vi "Klinger Control.vi"(8 "error in":errorcluster, 9 "PosDem":dbl caption="Allez à" min=-7999999.9 max=7999999.9 step=0.1 format="%.1f", 10 "Relatif":bool caption="Relatif/Absolu\n(Absolu)", 11 "Axe":u8(ring)=3 items=["W", "X", "Y", "Z"]) -> (0 "error out":errorcluster, 1 "Position":dbl min=-7999999.9 max=7999999.9 step=0.1 format="%.1f", 2 "NLimit":bool caption="Limite -", 3 "PLimit":bool caption="Limite +", 5 "Axe out":u8(ring)=3 caption="Axe" items=["W", "X", "Y", "Z"])   [LabVIEW 2010]
doc: "Ce Vi est une interface de contrôle complète d'où on peut effectué les diverse fonction du contrôlleur Klinger"
uses:
  <vilib>/Utility/error.llb/DialogType.ctl
  <userlib>/Klinger/Klinger Lib.llb/Klinger ConvUnitSgl.vi
  <userlib>/Klinger/Klinger Lib.llb/Klinger ConvUnitArr.vi
panel:
  in  "ReadPos":bool
  in  "ModParam":bool
  out "Nom de l'axe":string
  out "CorrParams":T1={"CorrActive"=FALSE, "ErreurLim"=0.1, "NbrEssais"=3} caption="Paramètres de \ncorrection de position" {"NbrEssais" min=1 max=5 step=1; "ErreurLim" min=0.0 max=10.0 step=0.1 format="%#.1f"}
  out "Adresse":string
  in  "Unit":u8(ring) caption="Unité:" items=["Pas", "mm", "ps", "Degré (°)"]
  in  "Default":bool
  in  "Zero":bool
  in  "Accel":sgl=0.4 caption="Accélération" min=0.1 max=2 step=0.1 format="%#.1f"
  in  "Speed Type":enum32{"Pas/Seconde", "ms/Pas"}(radio)
  in  "Vitesse":i32=800 min=32 max=4000 step=1 format="%#.0f"
  in  "stop":bool
  in  "RAZ":bool
  in  "Origine":bool
  out "PosErreur":dbl caption="Erreur de\nPositionnement" min=-7999999.9 max=7999999.9 step=0.1 format="%.1f"
  out "Indcomm":string caption="Terminal Indicateur"
  out "Pos Init":dbl caption="Position Initiale" min=-7999999.9 max=7999999.9 step=0.1 format="%.1f"
  out "Moving":bool caption="Déplacement\nen cours"
  out "Erreur":bool
  # "Commandes"
  # "Paramètres"
  # "Sec"
  # "Relatif"
  # "Absolu"
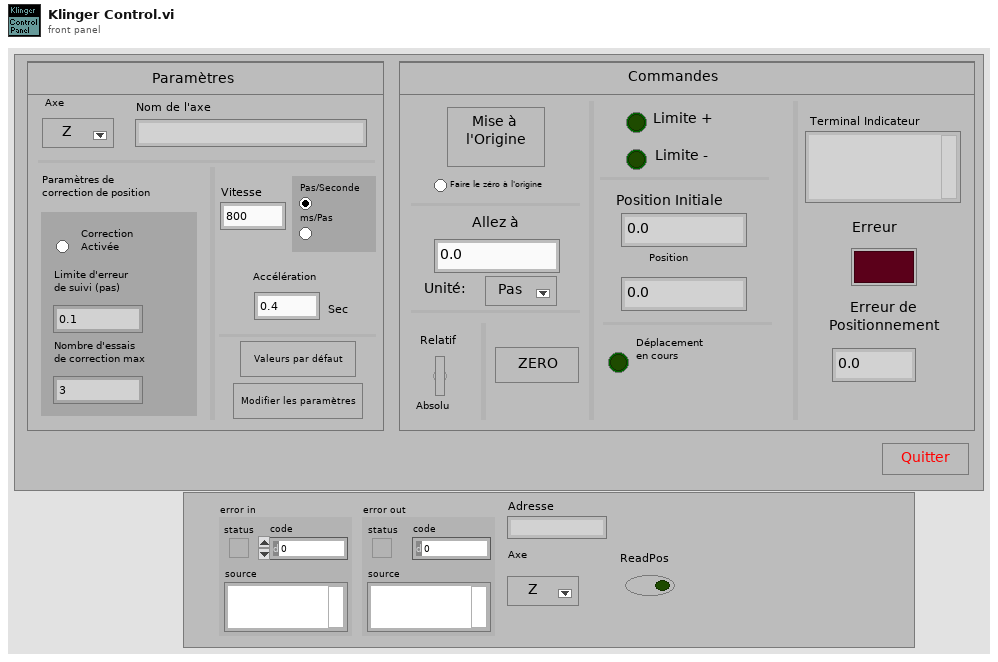
[diagram p1: front panel]
types:
  T1 = cluster{"CorrActive":bool, "ErreurLim":dbl, "NbrEssais":i32}
  T2 = cluster{"Minimum":dbl, "Maximum":dbl, "Increment":dbl}
  T3 = typedef "DialogType.ctl" = u16
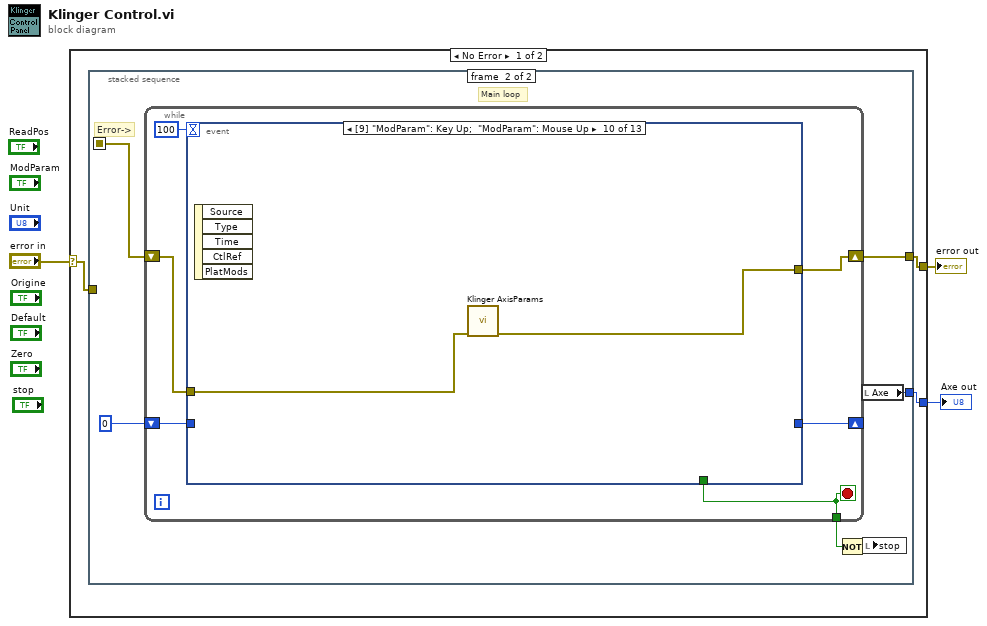
[diagram p0: block diagram]
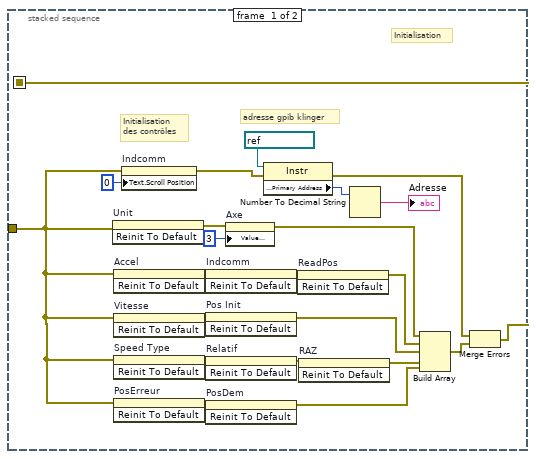
[diagram p2: hidden frame]
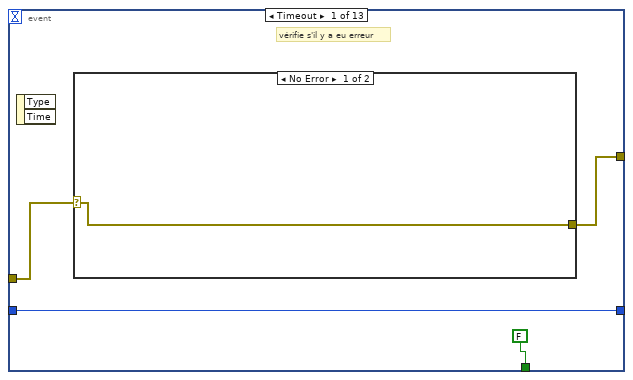
[diagram p3: hidden frame]
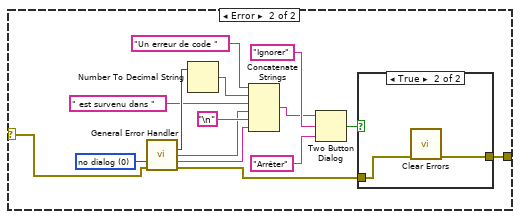
[diagram p4: hidden frame]
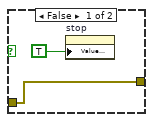
[diagram p5: hidden frame]
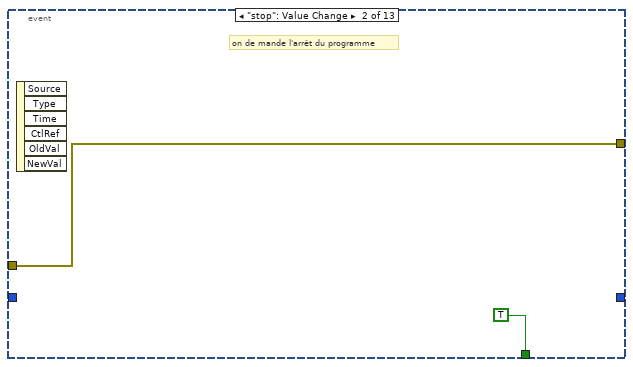
[diagram p6: hidden frame]
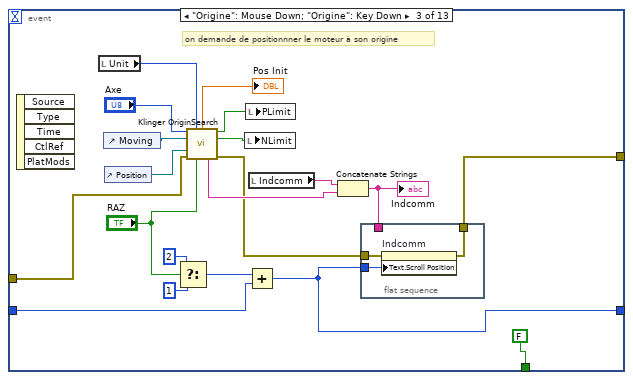
[diagram p7: hidden frame]
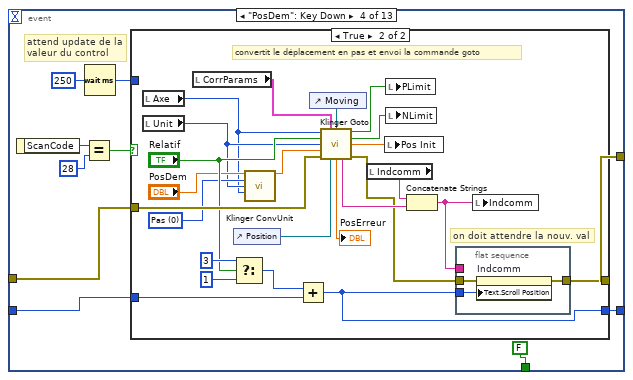
[diagram p8: hidden frame]
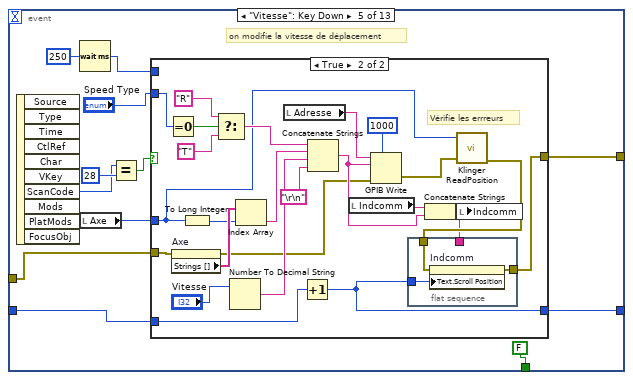
[diagram p10: hidden frame]
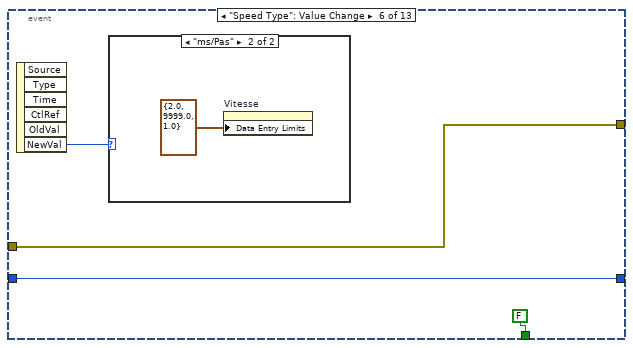
[diagram p12: hidden frame]
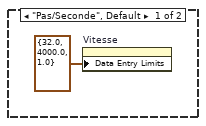
[diagram p13: hidden frame]
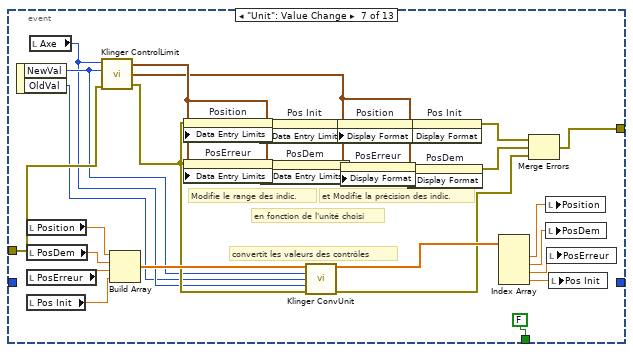
[diagram p14: hidden frame]
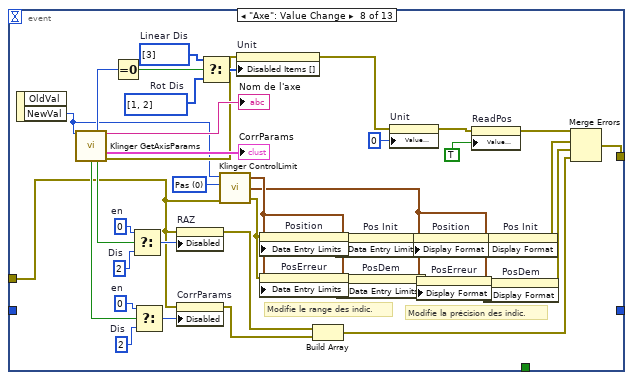
[diagram p15: hidden frame]
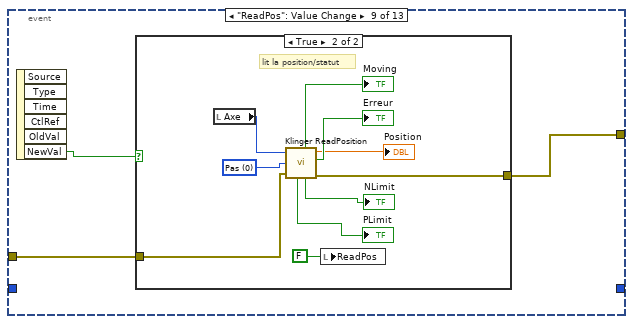
[diagram p16: hidden frame]
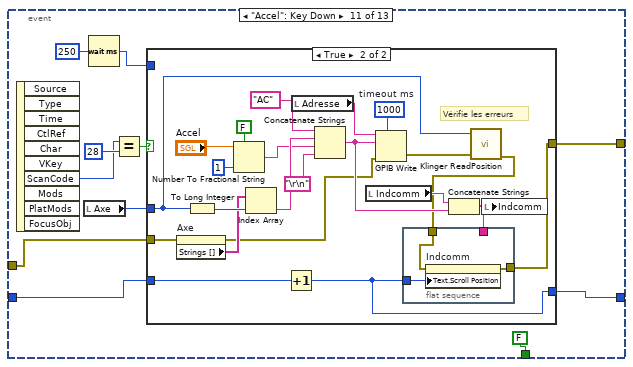
[diagram p18: hidden frame]
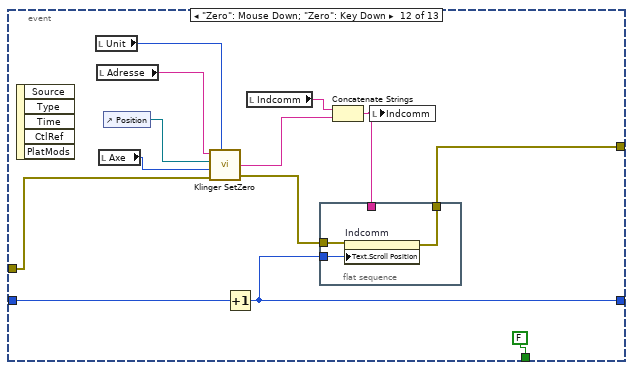
[diagram p20: hidden frame]
diagram:
  n1 = case shown="No Error" "error in" {
    selector: "error in" -> [w5 w345]
    tunnel: [w6 w345] -> w3
    tunnel: [w4 u8 0 ("Axe")] -> w1
    frame No Error {
      n2 = stacked-sequence {
        seq-local: [w7 _] -> [_ w33]
        tunnel: [_ w34] -> w6
        tunnel: w5 -> [w15 _]
        tunnel: [_ w29] -> w4
        frame #0 {
          # "adresse gpib klinger"
          # "Initialisation\ndes contrôles"
          # "Initialisation"
          n3 = invoke on="Unit" class="Ring (strict)" method="Reinit To Default"(error in=w15) -> (error out=w8:errorcluster)  [unwired: 2 in, 2 out]
          n4 = invoke on="Accel" class="DigNum (strict)" method="Reinit To Default"(error in=w15) -> (error out=w24:errorcluster)  [unwired: 2 in, 2 out]
          n5 = invoke on="Vitesse" class="DigNum (strict)" method="Reinit To Default"(error in=w15) -> (error out=w23:errorcluster)  [unwired: 2 in, 2 out]
          n6 = invoke on="Speed Type" class="RadioBtnsControl (strict)" method="Reinit To Default"(error in=w15) -> (error out=w22:errorcluster)  [unwired: 2 in, 2 out]
          n7 = invoke on="PosErreur" class="DigNum (strict)" method="Reinit To Default"(error in=w15) -> (error out=w17:errorcluster)  [unwired: 2 in, 2 out]
          n8 = property on="Indcomm" class="Str"(error in=w15, "Text.Scroll Position"=u32 0) -> (error out=w25:errorcluster)  [unwired: 1 in, 1 out]
          n9 = invoke on="Indcomm" class="Str" method="Reinit To Default"(error in=w24) -> (error out=w10:errorcluster)  [unwired: 2 in, 2 out]
          n10 = invoke on="Pos Init" class="DigNum (strict)" method="Reinit To Default"(error in=w23) -> (error out=w11:errorcluster)  [unwired: 2 in, 2 out]
          n11 = invoke on="Relatif" class="Bool (strict)" method="Reinit To Default"(error in=w22) -> (error out=w16:errorcluster)  [unwired: 2 in, 2 out]
          n12 = invoke on="PosDem" class="DigNum (strict)" method="Reinit To Default"(error in=w17) -> (error out=w21:errorcluster)  [unwired: 2 in, 2 out]
          n13 = property on="Axe" class="Ring (strict)"(error in=w8, "Value (Signaling)"=u8 3) -> (error out=w12:errorcluster)  [unwired: 1 in, 1 out]
          n14 = property class="Instr"(reference=refnum<visa-resource-name> "KLINGER", error in=w25) -> (error out=w19:errorcluster, "GPIB Settings:Primary Address"=w28:u16)  [unwired: 1 out]
          n15 = invoke on="ReadPos" class="Boolean (strict)" method="Reinit To Default"(error in=w10) -> (error out=w9:errorcluster)  [unwired: 2 in, 2 out]
          n16 = invoke on="RAZ" class="Bool (strict)" method="Reinit To Default"(error in=w16) -> (error out=w18:errorcluster)  [unwired: 2 in, 2 out]
          n17 = Number To Decimal String(number=w28) -> (decimal integer string=→"Adresse":string)  [unwired: 1 in]
          n18 = Build Array(w12, w9, w11, w18, w21) -> (w20:errorcluster[])
          n19 = Merge Errors(w19, w20) -> (w7:errorcluster)
        }
        frame #1 {
          # "Main loop"
          # "Error->"
          n20 = while {
            shift-right: [w36] -> w34
            shift-left: w33 -> [w39]
            shift-right: [w37] -> _
            shift-left: u32 0 ("Text.Scroll Position") -> [w38]
            tunnel: [w35] -> w31
            stop <- w35 stop-if-true
            n21 = event shown="[9] \"ModParam\": Key Up;  \"ModParam\": Mouse Up" {
              selector: _ -> [_ _ _ _ _ _ _ _ _ _ _ _ _]
              dyn-events: _ -> [_ _ _ _ _ _ _ _ _ _ _ _ _]
              timeout: 100 -> [_ _ _ _ _ _ _ _ _ _ _ _ _]
              tunnel: w39 -> [w41 w65 w77 w97 w136 w172 w188 w211 w244 w258 w266 w307 w334]
              tunnel: [w43 w65 w73 w93 w132 w172 w197 w217 w243 w257 w263 w300 w315] -> w36
              tunnel: w38 -> [w44 _ w82 w96 w135 w171 _ _ _ _ w262 w306 w331]
              tunnel: [w44 _ w81 w95 w134 w171 _ _ _ _ w265 w305 w317] -> w37
              tunnel: [FALSE TRUE FALSE FALSE FALSE FALSE FALSE _ _ _ FALSE FALSE FALSE] -> w35
              event Timeout {
                # "vérifie s'il y a eu erreur"
                n22 = event-data() -> ()  [unwired: 1 in, 2 out]
                n23 = case shown="No Error" w41 {
                  selector: w41 -> [w45 w46]
                  tunnel: [w45 w47] -> w43
                  frame No Error {
                  }
                  frame Error {
                    w57 = T3 0 items=["no dialog", "OK message", "continue or stop message", "OK message + warnings", "continue/stop + warnings"] ("type of dialog (OK msg:1)")
                    n24 = call <vilib>:"General Error Handler.vi"("type of dialog (OK msg:1)"=w57, "error in (no error)"=w46) -> ("code out"=w53:i32, "source out"=w52:string, "message"=w50:string, "error out"=w48:errorcluster)  [unwired: 9 in, 1 out]
                    n25 = Number To Decimal String(number=w53) -> (decimal integer string=w54:string)  [unwired: 1 in]
                    n26 = Concatenate Strings("Un erreur de code " ("string"), w54, " est survenu dans " ("string"), w52, "\n", w50) -> (w49:string)
                    n27 = Two Button Dialog(message=w49, 1:"Arrêter" ("F button name (\"Cancel\")"), 2:"Ignorer" ("T button name (\"OK\")")) -> (T button?=w60:bool)
                    n28 = case shown="True" w60 {
                      tunnel: w48 -> [w62 w64]
                      tunnel: [w62 w63] -> w47
                      frame False {
                        n29 = property on="stop" class="Bool (strict)"("Value (Signaling)"=TRUE) -> ()  [unwired: 2 in, 2 out]
                      }
                      frame True {
                        n30 = call <vilib>:"Clear Errors.vi"("error in (no error)"=w64) -> ("error out"=w63:errorcluster)  [unwired: 6 in]
                      }
                    }
                  }
                }
              }
              event "stop": Value Change {
                # "on de mande l'arrêt du programme"
                n31 = event-data() -> ()  [unwired: 1 in, 6 out]
              }
              event "Origine": Mouse Down; "Origine": Key Down {
                # "on demande de positionnner le moteur à son origine"
                n32 = event-data() -> ()  [unwired: 1 in, 5 out]
                n33 = local read "Unit"() -> (w67:u8)
                n34 = control-ref of="Moving"() -> (w83:refnum<vi>)
                n35 = control-ref of="Position"() -> (w84:refnum<vi>)
                n36 = Select(t=u32 2 ("x+y"), s="RAZ", f=u32 1 ("x+y")) -> (s? t:f=w80:u32)
                n37 = call <userlib>:"Klinger OriginSearch.vi"("Axe"="Axe", "UnitDem"=w67, "Moving Ref"=w83, "Position Ref"=w84, "error in"=w77, "Set as Zero"="RAZ") -> ("Pos Init"=→"Pos Init":dbl, "PLimit"=w85:bool, "NLimit"=w86:bool, "Indcomm"=w75:string, "error out"=w74:errorcluster)  [unwired: 3 in, 2 out]
                n38 = local write "NLimit"(w86) -> ()
                n39 = local write "PLimit"(w85) -> ()
                n40 = Add(x=w80, y=w82) -> (x+y=w81:u32)
                n41 = local read "Indcomm"() -> (w76:string)
                n42 = Concatenate Strings(w76, w75) -> (w69:string)
                "Indcomm" <- w69
                n43 = flat-sequence {
                  tunnel: w81 -> [w89]
                  tunnel: w69 -> [_]
                  tunnel: w74 -> [w88]
                  tunnel: [w87] -> w73
                  frame #0 {
                    n44 = property on="Indcomm" class="Str"(error in=w88, "Text.Scroll Position"=w89) -> (error out=w87:errorcluster)  [unwired: 1 in, 1 out]
                  }
                }
              }
              event "PosDem": Key Down {
                # "attend update de la \nvaleur du control"
                n45 = event-data() -> ("ScanCode"=w94:i16)  [unwired: 1 in]
                n46 = Equal?(x=w94, y=i16 28) -> (x = y?=w98:bool)
                n47 = Wait (ms)(milliseconds to wait=u32 250) -> (millisecond timer value=w91:u32)
                n48 = case shown="True" w98 {
                  tunnel: w97 -> [w100 w123]
                  tunnel: w96 -> [w101 w122]
                  tunnel: [w101 w113] -> w95
                  tunnel: [w100 w114] -> w93
                  tunnel: w91 -> [_ _]
                  frame False {
                  }
                  frame True {
                    w106 = u8 0 items=["Pas", "mm", "ps"] ("UnitDem")
                    # "convertit le déplacement en pas et envoi la commande goto"
                    # "on doit attendre la nouv. val"
                    n49 = local read "Axe"() -> (w103:u8)
                    n50 = local read "Unit"() -> (w104:u8)
                    n51 = local read "CorrParams"() -> (w102:T1)
                    n52 = control-ref of="Position"() -> (w115:refnum<vi>)
                    n53 = Select(t=u32 3 ("Text.Scroll Position"), s="Relatif", f=u32 1 ("Text.Scroll Position")) -> (s? t:f=w119:u32)
                    n54 = call-poly <userlib>:"Klinger ConvUnit.vi"("ParamAct"="PosDem", "UnitDem"=w106, "UnitAct"=w104, "Axe"=w103) -> ("ParamDem"=w105:dbl)  [unwired: 10 in, 1 out]
                    n55 = Add(x=w119, y=w122) -> (x+y=w113:u32)
                    n56 = control-ref of="Moving"() -> (w118:refnum<vi>)
                    n57 = call <userlib>:"Klinger Goto.vi"("Axe"=w103, "Suivi"=w102, "Moving Ref"=w118, "Relatif"="Relatif", "UnitDem"=w104, "PosDem"=w105, "error in"=w123, "Position Ref"=w115) -> ("PLimit"=w125:bool, "NLimit"=w124:bool, "Pos Init"=w109:dbl, "PosErreur"=→"PosErreur":dbl, "Indcomm"=w116:string, "error out"=w108:errorcluster)  [unwired: 2 out]
                    n58 = local read "Indcomm"() -> (w117:string)
                    n59 = local write "Pos Init"(w109) -> ()
                    n60 = local write "PLimit"(w125) -> ()
                    n61 = local write "NLimit"(w124) -> ()
                    n62 = Concatenate Strings(w117, w116) -> (w112:string)
                    n63 = flat-sequence {
                      tunnel: w113 -> [w128]
                      tunnel: w108 -> [w127]
                      tunnel: [w126] -> w114
                      tunnel: w112 -> [_]
                      frame #0 {
                        n64 = property on="Indcomm" class="Str"(error in=w127, "Text.Scroll Position"=w128) -> (error out=w126:errorcluster)  [unwired: 1 in, 1 out]
                      }
                    }
                    n65 = local write "Indcomm"(w112) -> ()
                  }
                }
              }
              event "Vitesse": Key Down {
                # "on modifie la vitesse de déplacement"
                n66 = event-data() -> ("ScanCode"=w133:i16)  [unwired: 1 in, 9 out]
                n67 = Wait (ms)(milliseconds to wait=u32 250) -> (millisecond timer value=w129:u32)
                n68 = local read "Axe"() -> (w137:u8)
                n69 = Equal?(x=w133, y=i16 28) -> (x = y?=w139:bool)
                n70 = case shown="True" w139 {
                  tunnel: "Speed Type" -> [_ w165]
                  tunnel: w137 -> [_ w148]
                  tunnel: [w142 w146] -> w132
                  tunnel: w136 -> [w142 w154]
                  tunnel: w135 -> [w141 w145]
                  tunnel: [w141 w153] -> w134
                  tunnel: w129 -> [_ _]
                  frame False {
                  }
                  frame True {
                    # "Vérifie les errreurs"
                    n71 = Equal To 0?(x=w165) -> (x = 0?=w164:bool)
                    n72 = property on="Axe" class="Ring (strict)"(error in=w154) -> (error out=w151:errorcluster, "Strings []"=w161:string[])  [unwired: 1 in, 1 out]
                    n73 = To Long Integer(number=w148) -> (32bit integer=w160:i32)
                    n74 = Select(t="R", s=w164, f="T") -> (s? t:f=w162:string)
                    n75 = Number To Decimal String(number="Vitesse") -> (decimal integer string=w157:string)  [unwired: 1 in]
                    n76 = Index Array(array=w161, index=w160) -> (element=w159:string)
                    n77 = local read "Adresse"() -> (w149:string)
                    n78 = Increment(x=w145) -> (x+1=w153:u32)
                    n79 = Concatenate Strings(w162, w159, w157, "\r\n") -> (w156:string)
                    n80 = local read "Indcomm"() -> (w155:string)
                    n81 = GPIB Write(0:w149, 1:w156, 3:w151, 4:1000 ("timeout ms (488.2 global)")) -> (6:w152:errorcluster)  [unwired: 1 in, 1 out]
                    n82 = flat-sequence {
                      tunnel: w153 -> [w169]
                      tunnel: w147 -> [w168]
                      tunnel: [w167] -> w146
                      tunnel: w144 -> [_]
                      frame #0 {
                        n83 = property on="Indcomm" class="Str"(error in=w168, "Text.Scroll Position"=w169) -> (error out=w167:errorcluster)  [unwired: 1 in, 1 out]
                      }
                    }
                    n84 = Concatenate Strings(w155, w156) -> (w144:string)
                    n85 = call <userlib>:"Klinger ReadPosition.vi"("Axe"=w148, "error in"=w152) -> ("error out"=w147:errorcluster)  [unwired: 2 in, 6 out]
                    n86 = local write "Indcomm"(w144) -> ()
                  }
                }
              }
              event "Speed Type": Value Change {
                n87 = event-data() -> ("NewVal"=w173:enum32{"Pas/Seconde", "ms/Pas"})  [unwired: 1 in, 5 out]
                n88 = case shown="\"ms/Pas\"" w173 {
                  frame "Pas/Seconde", Default {
                    n89 = property on="Vitesse" class="DigNum (strict)"("Data Entry Limits"=T2 {"Minimum"=32.0, "Maximum"=4000.0, "Increment"=1.0} ("Data Range")) -> ()  [unwired: 2 in, 2 out]
                  }
                  frame "ms/Pas" {
                    n90 = property on="Vitesse" class="DigNum (strict)"("Data Entry Limits"=T2 {"Minimum"=2.0, "Maximum"=9999.0, "Increment"=1.0} ("Data Range")) -> ()  [unwired: 2 in, 2 out]
                  }
                }
              }
              event "Unit": Value Change {
                # "convertit les valeurs des contrôles"
                # "en fonction de l'unité choisi"
                # "et Modifie la précision des indic."
                # "Modifie le range des indic."
                n91 = event-data() -> ("NewVal"=w178:u8, "OldVal"=w176:u8)  [unwired: 1 in]
                n92 = local read "Position"() -> (w201:dbl)
                n93 = local read "PosDem"() -> (w202:dbl)
                n94 = local read "PosErreur"() -> (w203:dbl)
                n95 = local read "Pos Init"() -> (w200:dbl)
                n96 = local read "Axe"() -> (w177:u8)
                n97 = call <userlib>:"Klinger ControlLimit.vi"("Axe"=w177, "UnitDem"=w178, "error in"=w188) -> ("DataRange"=w186:T2, "FormtPrec"=w185:cluster{"Format":u8, "Precision":u8}, "error out"=w187:errorcluster)  [unwired: 2 in]
                n98 = Build Array(w201, w202, w203, w200) -> (w195:dbl[])
                n99 = property on="Position" class="DigNum (strict)"(error in=w187, "Data Entry Limits"=w186) -> (error out=w184:errorcluster)  [unwired: 1 in, 1 out]
                n100 = property on="PosErreur" class="DigNum (strict)"(error in=w187, "Data Entry Limits"=w186) -> (error out=w183:errorcluster)  [unwired: 1 in, 1 out]
                n101 = property on="Pos Init" class="DigNum (strict)"(error in=w184, "Data Entry Limits"=w186) -> (error out=w179:errorcluster)  [unwired: 1 in, 1 out]
                n102 = property on="PosDem" class="DigNum (strict)"(error in=w183, "Data Entry Limits"=w186) -> (error out=w180:errorcluster)  [unwired: 1 in, 1 out]
                n103 = call-poly <userlib>:"Klinger ConvUnit.vi"("ParamAct"=w195, "UnitDem"=w178, "UnitAct"=w176, "Axe"=w177, "error in"=w187) -> ("ParamDem"=w194:dbl[], "error out"=w189:errorcluster)  [unwired: 9 in]
                n104 = property on="Position" class="DigNum (strict)"(error in=w179, "Display Format"=w185) -> (error out=w182:errorcluster)  [unwired: 1 in, 1 out]
                n105 = property on="PosErreur" class="DigNum (strict)"(error in=w180, "Display Format"=w185) -> (error out=w181:errorcluster)  [unwired: 1 in, 1 out]
                n106 = property on="Pos Init" class="DigNum (strict)"(error in=w182, "Display Format"=w185) -> (error out=w199:errorcluster)  [unwired: 1 in, 1 out]
                n107 = property on="PosDem" class="DigNum (strict)"(error in=w181, "Display Format"=w185) -> (error out=w198:errorcluster)  [unwired: 1 in, 1 out]
                n108 = Index Array(array=w194) -> (element #1=w193:dbl, element #2=w192:dbl, element #3=w191:dbl, element #4=w190:dbl)  [unwired: 4 in]
                n109 = Merge Errors(w199, w198, w189) -> (w197:errorcluster)
                n110 = local write "Position"(w193) -> ()
                n111 = local write "PosDem"(w192) -> ()
                n112 = local write "PosErreur"(w191) -> ()
                n113 = local write "Pos Init"(w190) -> ()
              }
              event "Axe": Value Change {
                w218 = u8 0 items=["Pas", "mm", "ps", "Degré (°)"] ("UnitDem")
                w231 = i32[] [1, 2]  # Rot Dis
                w232 = i32[] [3]  # Linear Dis
                w236 = u8 2  # Dis
                w235 = u8 0  # en
                w238 = u8 2  # Dis
                w239 = u8 0  # en
                # "Modifie la précision des indic."
                # "Modifie le range des indic."
                n114 = event-data() -> ("NewVal"=w209:u8)  [unwired: 1 in, 1 out]
                n115 = call <userlib>:"Klinger GetAxisParams.vi"("Axe"=w209) -> ("TypeMouv"=w230:i32, "Nom de l'axe"=→"Nom de l'axe":string, "CorrParams"=→"CorrParams":T1, "Encodeur"=w237:bool, "MiseàZéro"=w234:bool, "error out"=w210:errorcluster)  [unwired: 7 in, 2 out]
                n116 = Equal To 0?(x=w230) -> (x = 0?=w229:bool)
                n117 = Select(t=w235, s=w234, f=w236) -> (s? t:f=w233:u8)
                n118 = Select(t=w239, s=w237, f=w238) -> (s? t:f=w240:u8)
                n119 = property on="RAZ" class="Bool (strict)"(error in=w211, "Disabled"=w233) -> (error out=w216:errorcluster)  [unwired: 1 in, 1 out]
                n120 = property on="CorrParams" class="Clust (strict)"(error in=w211, "Disabled"=w240) -> (error out=w215:errorcluster)  [unwired: 1 in, 1 out]
                n121 = Select(t=w232, s=w229, f=w231) -> (s? t:f=w228:i32[])
                n122 = call <userlib>:"Klinger ControlLimit.vi"("Axe"=w209, "UnitDem"=w218, "error in"=w211) -> ("DataRange"=w227:T2, "FormtPrec"=w226:cluster{"Format":u8, "Precision":u8}, "error out"=w219:errorcluster)  [unwired: 2 in]
                n123 = property on="Unit" class="Ring (strict)"(error in=w210, "Disabled Items []"=w228) -> (error out=w207:errorcluster)  [unwired: 1 in, 1 out]
                n124 = property on="Position" class="DigNum (strict)"(error in=w219, "Data Entry Limits"=w227) -> (error out=w225:errorcluster)  [unwired: 1 in, 1 out]
                n125 = property on="PosErreur" class="DigNum (strict)"(error in=w219, "Data Entry Limits"=w227) -> (error out=w224:errorcluster)  [unwired: 1 in, 1 out]
                n126 = Build Array(w216, w215) -> (w212:errorcluster[])
                n127 = property on="Pos Init" class="DigNum (strict)"(error in=w225, "Data Entry Limits"=w227) -> (error out=w220:errorcluster)  [unwired: 1 in, 1 out]
                n128 = property on="PosDem" class="DigNum (strict)"(error in=w224, "Data Entry Limits"=w227) -> (error out=w221:errorcluster)  [unwired: 1 in, 1 out]
                n129 = property on="Unit" class="Ring (strict)"(error in=w207, "Value (Signaling)"=u8 0) -> (error out=w206:errorcluster)  [unwired: 1 in, 1 out]
                n130 = property on="Position" class="DigNum (strict)"(error in=w220, "Display Format"=w226) -> (error out=w223:errorcluster)  [unwired: 1 in, 1 out]
                n131 = property on="PosErreur" class="DigNum (strict)"(error in=w221, "Display Format"=w226) -> (error out=w222:errorcluster)  [unwired: 1 in, 1 out]
                n132 = property on="ReadPos" class="Bool (strict)"(error in=w206, "Value (Signaling)"=TRUE) -> (error out=w204:errorcluster)  [unwired: 1 in, 1 out]
                n133 = property on="Pos Init" class="DigNum (strict)"(error in=w223, "Display Format"=w226) -> (error out=w213:errorcluster)  [unwired: 1 in, 1 out]
                n134 = property on="PosDem" class="DigNum (strict)"(error in=w222, "Display Format"=w226) -> (error out=w214:errorcluster)  [unwired: 1 in, 1 out]
                n135 = Merge Errors(w204, w213, w214, w212) -> (w217:errorcluster)
              }
              event "ReadPos": Value Change {
                n136 = event-data() -> ("NewVal"=w245:bool)  [unwired: 1 in, 5 out]
                n137 = case shown="True" w245 {
                  tunnel: w244 -> [w246 w254]
                  tunnel: [w246 w253] -> w243
                  frame False {
                  }
                  frame True {
                    w256 = u8 0 items=["Pas", "mm", "ps", "Degré (°)"] ("UnitDem")
                    # "lit la position/statut"
                    n138 = local read "Axe"() -> (w255:u8)
                    n139 = call <userlib>:"Klinger ReadPosition.vi"("Axe"=w255, "UnitDem"=w256, "error in"=w254) -> ("PLimit"=→"PLimit":bool, "Moving"=→"Moving":bool, "Position"=→"Position":dbl, "Statut"=→"Erreur":bool, "NLimit"=→"NLimit":bool, "error out"=w253:errorcluster)  [unwired: 1 in, 1 out]
                    n140 = local write "ReadPos"(FALSE ("ReadPos")) -> ()
                  }
                }
              }
              event "ModParam": Key Up; "ModParam": Mouse Up {
                n141 = event-data() -> ()  [unwired: 1 in, 5 out]
                n142 = call <userlib>:"Klinger AxisParams.vi"("error in"=w258) -> ("error out"=w257:errorcluster)  [unwired: 14 in]
              }
              event "Accel": Key Down {
                n143 = event-data() -> ("ScanCode"=w264:i16)  [unwired: 1 in, 9 out]
                n144 = local read "Axe"() -> (w267:u8)
                n145 = Wait (ms)(milliseconds to wait=u32 250) -> (millisecond timer value=w260:u32)
                n146 = Equal?(x=w264, y=i16 28) -> (x = y?=w268:bool)
                n147 = case shown="True" w268 {
                  tunnel: w267 -> [_ w280]
                  tunnel: w266 -> [w270 w286]
                  tunnel: w262 -> [w271 w277]
                  tunnel: [w271 w276] -> w265
                  tunnel: [w270 w274] -> w263
                  tunnel: w260 -> [_ _]
                  frame False {
                  }
                  frame True {
                    w278 = 1000  # timeout ms
                    # "Vérifie les erreurs"
                    n148 = property on="Axe" class="Ring (strict)"(error in=w286) -> (error out=w283:errorcluster, "Strings []"=w289:string[])  [unwired: 1 in, 1 out]
                    n149 = To Long Integer(number=w280) -> (32bit integer=w292:i32)
                    n150 = Number To Fractional String(use system decimal point (T)=FALSE, number="Accel", precision (6)=i16 1) -> (F-format string=w288:string)  [unwired: 1 in]
                    n151 = Index Array(array=w289, index=w292) -> (element=w291:string)
                    n152 = Increment(x=w277) -> (x+1=w276:u32)
                    n153 = local read "Adresse"() -> (w279:string)
                    n154 = Concatenate Strings("AC" ("string"), w291, w288, "\r\n") -> (w284:string)
                    n155 = local read "Indcomm"() -> (w285:string)
                    n156 = GPIB Write(0:w279, 1:w284, 3:w283, 4:w278) -> (6:w281:errorcluster)  [unwired: 1 in, 1 out]
                    n157 = flat-sequence {
                      tunnel: w276 -> [w296]
                      tunnel: w275 -> [_]
                      tunnel: [w295] -> w274
                      tunnel: w273 -> [w294]
                      frame #0 {
                        n158 = property on="Indcomm" class="Str"(error in=w294, "Text.Scroll Position"=w296) -> (error out=w295:errorcluster)  [unwired: 1 in, 1 out]
                      }
                    }
                    n159 = Concatenate Strings(w285, w284) -> (w275:string)
                    n160 = call <userlib>:"Klinger ReadPosition.vi"("Axe"=w280, "error in"=w281) -> ("error out"=w273:errorcluster)  [unwired: 2 in, 6 out]
                    n161 = local write "Indcomm"(w275) -> ()
                  }
                }
              }
              event "Zero": Mouse Down; "Zero": Key Down {
                n162 = event-data() -> ()  [unwired: 1 in, 5 out]
                n163 = local read "Unit"() -> (w297:u8)
                n164 = local read "Adresse"() -> (w302:string)
                n165 = local read "Axe"() -> (w309:u8)
                n166 = control-ref of="Position"() -> (w308:refnum<vi>)
                n167 = call <userlib>:"Klinger SetZero.vi"("Address GPIB"=w302, "Position Ref"=w308, "Axe"=w309, "error in"=w307, "UnitDem"=w297) -> ("Ind Comm"=w303:string, "error out"=w301:errorcluster)  [unwired: 1 out]
                n168 = Increment(x=w306) -> (x+1=w305:u32)
                n169 = local read "Indcomm"() -> (w304:string)
                n170 = flat-sequence {
                  tunnel: w305 -> [w312]
                  tunnel: w301 -> [w311]
                  tunnel: [w310] -> w300
                  tunnel: w299 -> [_]
                  frame #0 {
                    n171 = property on="Indcomm" class="Str"(error in=w311, "Text.Scroll Position"=w312) -> (error out=w310:errorcluster)  [unwired: 1 in, 1 out]
                  }
                }
                n172 = Concatenate Strings(w304, w303) -> (w299:string)
                n173 = local write "Indcomm"(w299) -> ()
              }
              event "Default": Key Down; "Default": Mouse Down {
                w320 = 1000  # timeout ms
                w327 = "800" ("string")
                w323 = "0.4" ("string")
                w335 = "\r\n"
                n174 = event-data() -> ()  [unwired: 1 in, 5 out]
                n175 = local read "Axe"() -> (w319:u8)
                n176 = property on="Axe" class="Ring (strict)"(error in=w334) -> (error out=w333:errorcluster, "Strings []"=w339:string[])  [unwired: 1 in, 1 out]
                n177 = To Long Integer(number=w319) -> (32bit integer=w340:i32)
                n178 = Index Array(array=w339, index=w340) -> (element=w336:string)
                n179 = local write "Speed Type"(enum32{"Pas/Seconde", "ms/Pas"}."Pas/Seconde" ("Speed Type")) -> ()
                n180 = local read "Adresse"() -> (w321:string)
                n181 = Decimal String To Number(string=w327) -> (number=w326:i32)  [unwired: 2 in, 1 out]
                n182 = Concatenate Strings("AC" ("data"), w336, w323, w335, "R" ("data"), w336, w327, w335) -> (w330:string)
                n183 = property on="Vitesse" class="DigNum (strict)"("Value"=w326) -> ()  [unwired: 2 in, 2 out]
                n184 = GPIB Write(0:w321, 1:w330, 3:w333, 4:w320) -> (6:w322:errorcluster)  [unwired: 1 in, 1 out]
                n185 = local read "Indcomm"() -> (w332:string)
                n186 = Fract/Exp String To Number(use system decimal point (T)=FALSE, string=w323, default (0 dbl)=sgl 0.0) -> (number=w328:sgl)  [unwired: 1 in, 1 out]
                n187 = Add(x=u32 2, y=w331) -> (x+y=w317:u32)
                n188 = property on="Accel" class="DigNum (strict)"("Value"=w328) -> ()  [unwired: 2 in, 2 out]
                n189 = Concatenate Strings(w332, w330) -> (w318:string)
                n190 = flat-sequence {
                  tunnel: w317 -> [w343]
                  tunnel: w318 -> [_]
                  tunnel: w316 -> [w342]
                  tunnel: [w341] -> w315
                  frame #0 {
                    n191 = property on="Indcomm" class="Str"(error in=w342, "Text.Scroll Position"=w343) -> (error out=w341:errorcluster)  [unwired: 1 in, 1 out]
                  }
                }
                n192 = call <userlib>:"Klinger ReadPosition.vi"("Axe"=w319, "error in"=w322) -> ("error out"=w316:errorcluster)  [unwired: 2 in, 6 out]
                n193 = local write "Indcomm"(w318) -> ()
              }
            }
          }
          n194 = Not(x=w31) -> (.not. x?=w30:bool)
          n195 = local read "Axe"() -> (w29:u8)
          n196 = local write "stop"(w30) -> ()
        }
      }
    }
    frame Error {
    }
  }
  "error out" <- w3
  "Axe out" <- w1
